vi "Initialize Daemon.vi"(8 "error in (no error)":errorcluster, 9 "data model":refnum<class "Device Data Model.lvclass">, 10 "transmission data unit":refnum<class "Transmission Data Unit.lvclass">, 11 "network slave in":refnum<class "Network Slave.lvclass">) -> (0 "error out":errorcluster, 3 "network slave out":refnum<class "Network Slave.lvclass">)   [LabVIEW 2017, in "SubVIs.lvlib" / "Network Slave.lvclass"]
doc: "This provides an interface for the slave to launch a protocol daemon."
uses:
  <vilib>/Modbus/subvis/Protocol/Interfaces/Network Slave/Network Slave.lvclass
  <vilib>/Modbus/subvis/Transmission Data Unit (ADU)/Transmission Data Unit/Transmission Data Unit.lvclass
  <vilib>/Modbus/subvis/Data and Functions/Device Data Model/Device Data Model.lvclass
  <vilib>/Modbus/subvis/Protocol/Interfaces/Network Slave/Network Slave.lvclass/Network Slave.ctl
  <vilib>/Modbus/subvis/SubVIs.lvlib
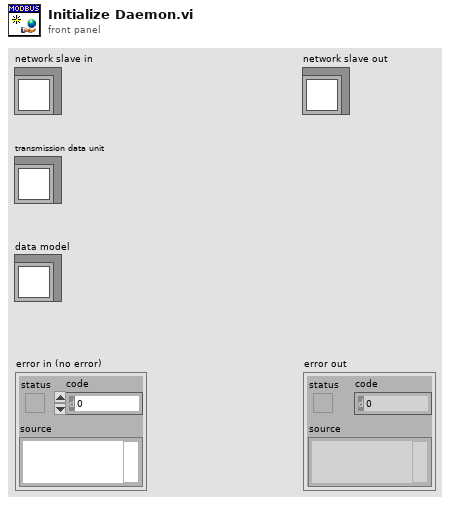
[diagram p1: front panel]
types:
  T1 = cluster{"error":errorcluster, "status":enum16{"Not Started", "Running", "Error", "Stopped"}}
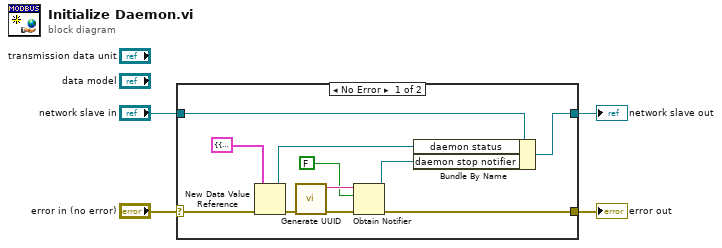
[diagram p0: block diagram]
diagram:
  n1 = case shown="No Error" "error in (no error)" {
    selector: "error in (no error)" -> [w11 w16]
    tunnel: "network slave in" -> [w14 w15]
    tunnel: [w13 w15] -> w3
    tunnel: [w8 w16] -> w1
    frame No Error {
      n2 = New Data Value Reference(data value=T1 {"error"={"status"=FALSE, "code"=0, "source"=""}, "status"=enum."Not Started"} ("Status"), error in=w11) -> (data value reference=w12:refnum<data-value>, error out=w9:errorcluster)
      n3 = call <vilib>:"Generate UUID.vi"() -> ("UUID"=w7:string)  [unwired: 11 in]
      n4 = Obtain Notifier(name (unnamed)=w7, notification data type=FALSE, error in (no error)=w9) -> (notifier out=w5:refnum<notifier>, error out=w8:errorcluster)  [unwired: 1 in, 1 out]
      n5 = Bundle By Name(cluster=w14, "daemon status"=w12, "daemon stop notifier"=w5) -> (w13:refnum<class "Network Slave.lvclass">)
    }
    frame Error {
    }
  }
  "error out" <- w1
  "network slave out" <- w3
